vi "Fetch the IO Controls.vi"(0 "vi path":path, 11 "error in":errorcluster) -> (4 "io controls[]":string[](array[string]), 15 "error out":errorcluster)   [LabVIEW 2021, in "Converter.lvlib"]
uses:
  Converter.lvlib
  Converter Reusables/Converter Reusables.lvlib
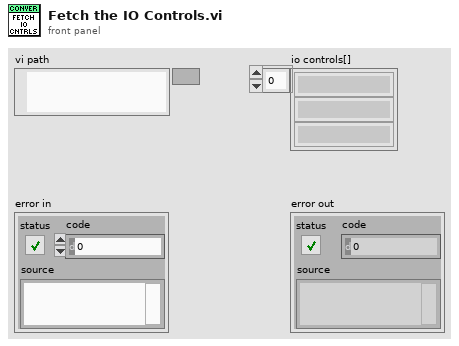
[diagram p1: front panel]
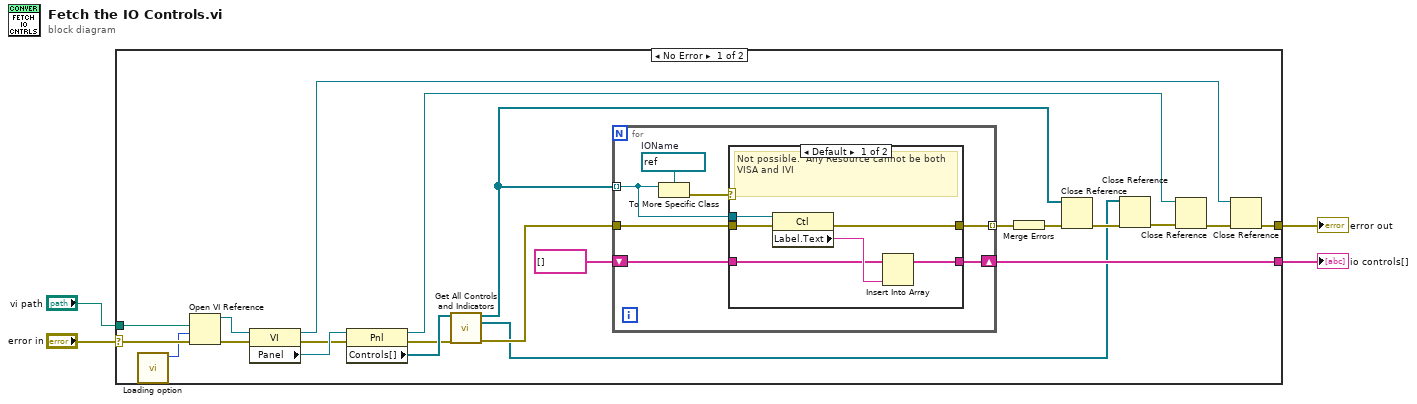
[diagram p0: block diagram]
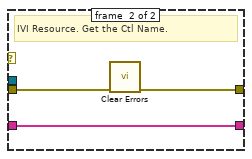
[diagram p2: hidden frame]
diagram:
  n1 = case shown="No Error" "error in" {
    selector: "error in" -> [w17 w43]
    tunnel: [w20 _] -> w1
    tunnel: [w16 w43] -> w3
    tunnel: "vi path" -> [w15 _]
    frame No Error {
      n2 = call "Loading option.vi"() -> ("options"=w5:i32)  [unwired: 11 in]
      n3 = Open VI Reference(vi path=w15, options=w5, error in (no error)=w17) -> (vi reference=w26:refnum<vi>, error out=w24:errorcluster)  [unwired: 3 in]
      n4 = property class="VI"(reference=w26, error in=w24) -> (reference out=w18:refnum<vi>, error out=w23:errorcluster, "Panel"=w25:refnum<vi>)
      n5 = property class="Pnl"(reference=w25, error in=w23) -> (reference out=w7:refnum<vi>, error out=w12:errorcluster, "Controls[]"=w14:refnum<vi>[])
      n6 = call "Get All Controls and Indicators.vi"("controls[]"=w14, "error in"=w12) -> ("controls[]"=w11:refnum<vi>[], "indicators[]"=w8:refnum<vi>[], "error out"=w13:errorcluster)  [unwired: 11 in]
      n7 = for {
        tunnel: w11 -> [w27] mode=indexing
        tunnel: w13 -> [w33]
        tunnel: [w32] -> w22 mode=indexing
        shift-right: [w30] -> w20
        shift-left: string[] [] -> [w31]
        w28 = refnum<vi> refnum  # IOName
        n8 = To More Specific Class(target class=w28, reference=w27) -> (error out=w29:errorcluster)  [unwired: 1 in, 1 out]
        n9 = case shown="Default" w29 {
          tunnel: w27 -> [w37 _]
          tunnel: [w36 w40] -> w32
          tunnel: w33 -> [w38 w42]
          tunnel: w31 -> [w34 w41]
          tunnel: [w35 w41] -> w30
          frame #0 {
            # "Not possible.  Any Resource cannot be both VISA and IVI"
            n10 = property class="Ctl"(reference=w37, error in=w38) -> (error out=w36:errorcluster, "Label.Text"=w39:string)  [unwired: 1 out]
            n11 = Insert Into Array(array=w34, new element=w39) -> (w35:string[])  [unwired: 1 in]
          }
          frame #1 {
            # "IVI Resource. Get the Ctl Name."
            n12 = call <vilib>:"Clear Errors.vi"("error in (no error)"=w42) -> ("error out"=w40:errorcluster)  [unwired: 5 in, 1 out]
          }
        }
      }
      n13 = Merge Errors(w22) -> (w21:errorcluster)
      n14 = Close Reference(reference=w11, error in (no error)=w21) -> (error out=w10:errorcluster)
      n15 = Close Reference(reference=w8, error in (no error)=w10) -> (error out=w9:errorcluster)
      n16 = Close Reference(reference=w7, error in (no error)=w9) -> (error out=w19:errorcluster)
      n17 = Close Reference(reference=w18, error in (no error)=w19) -> (error out=w16:errorcluster)
    }
    frame Error {
    }
  }
  "error out" <- w3
  "io controls[]" <- w1
